vi "Configure Multi Eval Meas Symbol Rate Error Limit.vi"(7 "Symbol Rate (On)":bool=TRUE, 8 "error in (no error)":errorcluster, 9 "Symbol Rate (0)":dbl format="%^.3e", 10 "Instance (1)":i32=1, 11 "VISA resource name":refnum<visa-resource-name>) -> (0 "error out":errorcluster, 3 "VISA resource name out":refnum<visa-resource-name>)   [LabVIEW 2020, in "Rohde&Schwarz CMP LR WPAN Measurement.lvlib"]
doc: "Defines upper limit for symbol rate error.\n\nOrder of parameters:\n<SymbolRate>\n<SymbolRateEnble> - Disables | enables the limit check for symbol rate error.\n\nAttribute:\n-\n\nRemote-control command:\nCONFigure:WPAN:MEAS<i>:MEValuation:LIMit:SRATe"
uses:
  <instrlib>/Rohde&Schwarz CMP LR WPAN Measurement/Rohde&Schwarz CMP LR WPAN Measurement.lvlib
  <instrlib>/Rohde&Schwarz CMP LR WPAN Measurement/Private/rsidr_core.llb/rsidr_core.lvlib
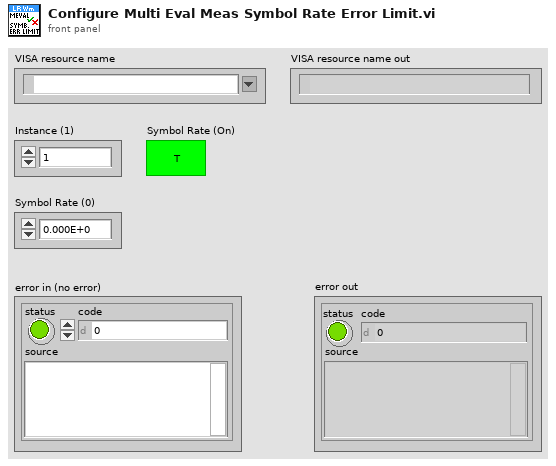
[diagram p1: front panel]
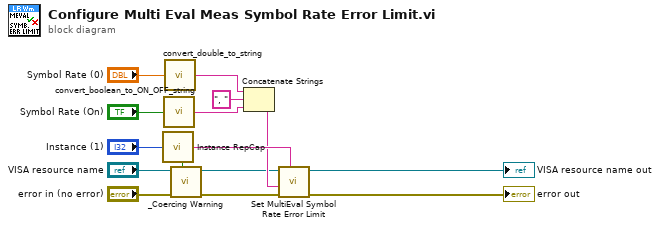
[diagram p0: block diagram]
diagram:
  n1 = call <instrlib>:"Instance RepCap.vi"("Instance In"="Instance (1)") -> ("In Range?"=w15:bool, "RepCap Identifier Out"=w14:string)  [unwired: 1 in]
  n2 = call <instrlib>:"convert_boolean_to_ON_OFF_string.vi"("boolean value in"="Symbol Rate (On)") -> ("string value out"=w9:string)  [unwired: 4 in]
  n3 = call <instrlib>:"convert_double_to_string.vi"("double in"="Symbol Rate (0)") -> ("string out"=w10:string)  [unwired: 4 in]
  n4 = call <instrlib>:"_Coercing Warning.vi"("In Range?"=w15, "error in (no error)"="error in (no error)", "VISA resource name"="VISA resource name") -> ("error out"=w5:errorcluster, "VISA resource name out"=w4:refnum<visa-resource-name>)  [unwired: 7 in]
  n5 = Concatenate Strings(w10, ", " ("string"), w9) -> (w8:string)
  n6 = call "Set MultiEval Symbol Rate Error Limit"("Repeated Capabilities"=w14, "error in (no error)"=w5, "MultiEval Symbol Rate Error Limit ()"=w8, "instrument handle"=w4) -> ("error out"=→"error out":errorcluster, "instrument handle out"=→"VISA resource name out":refnum<visa-resource-name>)  [unwired: 6 in]
